vi "example-VariantClusterAccessMulti.vi"() -> ()   [LabVIEW 2020]
panel:
  out "Old Values":variant[](array[variant])
  out "Revised Cluster":variant
  in  "New Values":variant[](array[variant])
  in  "Labels":string[](array[string])
  in  "Cluster":variant
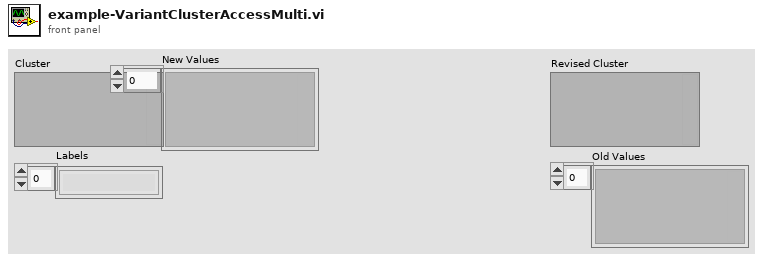
[diagram p1: front panel]
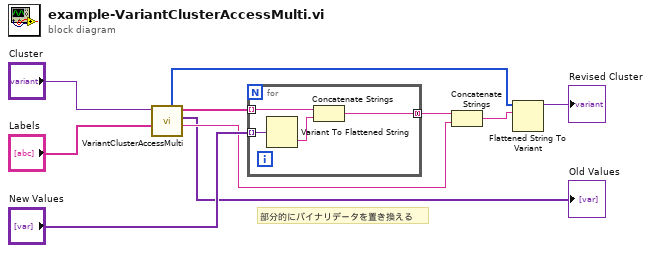
[diagram p0: block diagram]
diagram:
  # "部分的にバイナリデータを置き換える"
  n1 = call "VariantClusterAccessMulti.vi"("labels"="Labels", "Value in"="Cluster") -> ("rest"=w5:string, "values"=→"Old Values":variant[], "prepends"=w8:string[], "type string"=w3:i16[])  [unwired: 5 in, 1 out]
  n2 = for {
    tunnel: w8 -> [w13] mode=indexing
    tunnel: "New Values" -> [w14] mode=indexing
    tunnel: [w11] -> w6 mode=concatenating
    n3 = Variant To Flattened String(Variant=w14) -> (data string=w12:string)  [unwired: 1 out]
    n4 = Concatenate Strings(w13, w12) -> (w11:string)
  }
  n5 = Concatenate Strings(w6, w5) -> (w4:string)
  n6 = Flattened String To Variant(6:w4, 7:w3) -> (3:→"Revised Cluster":variant)  [unwired: 1 in, 1 out]
